vi "sub_pwrpak7_data-check.vi"() -> ()   [LabVIEW 2019]
panel:
  out "heading":dbl
  out "heading_check":bool
  out "heading_str":string
  out "index":i32
  out "경도":string="126.72082016226"
  out "위도":string="37.37012814476"
  out "utm-1":cluster{dbl, dbl}={530126.7583503594, 175270.68061157822} {"?" format="%#.6f"; "?" format="%.6f"}
  out "wgs84-1":cluster{dbl, dbl}={126.72082016226, 37.37012814476}
  in  "gps receive parsing array":string[](array[string])
  out "mode check":bool
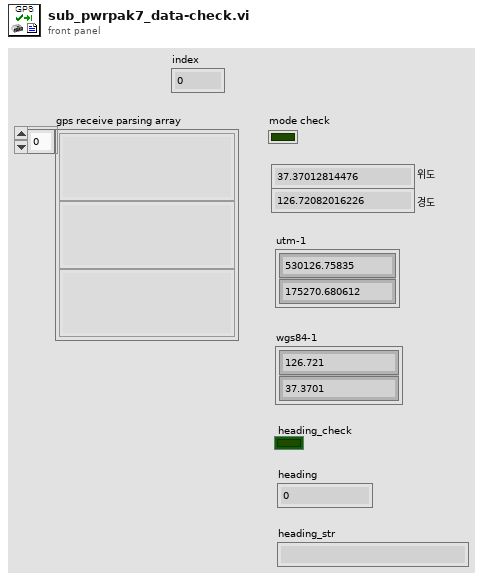
[diagram p1: front panel]
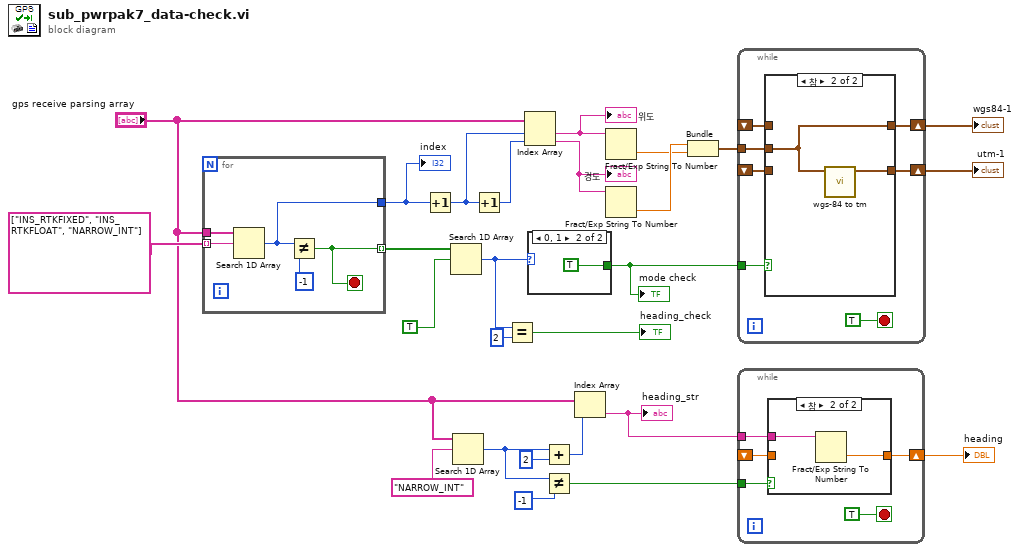
[diagram p0: block diagram]
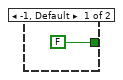
[diagram p2: hidden frame]
diagram:
  n1 = for {
    tunnel: [w28] -> w7 mode=indexing
    tunnel: "gps receive parsing array" -> [w31]
    tunnel: string[] ["INS_RTKFIXED", "INS_RTKFLOAT", "NARROW_INT"] -> [w29] mode=indexing
    tunnel: [w27] -> w17
    stop <- w28 stop-if-true
    n2 = Search 1D Array(1D array=w31, element=w29) -> (index of element=w27:i32)  [unwired: 1 in]
    n3 = Not Equal?(x=w27, y=-1) -> (x != y?=w28:bool)
  }
  "index" <- w17
  n4 = Increment(x=w17) -> (x+1=w21:i32)
  n5 = Search 1D Array(1D array=w7, element=TRUE ("원소")) -> (index of element=w3:i32)  [unwired: 1 in]
  n6 = Search 1D Array(1D array="gps receive parsing array", element="NARROW_INT" ("원소")) -> (index of element=w13:i32)  [unwired: 1 in]
  n7 = Increment(x=w21) -> (x+1=w20:i32)
  n8 = Equal?(x=w3, y=2) -> (x = y?=→"heading_check":bool)
  n9 = Index Array(array="gps receive parsing array", index #1=w21, index #2=w20) -> (element #1=w26:string, element #2=w25:string)
  "위도" <- w26
  "경도" <- w25
  n10 = case shown="0, 1" w3 {
    tunnel: [FALSE TRUE] -> w2
    frame -1, Default {
    }
    frame 0, 1 {
    }
  }
  "mode check" <- w2
  n11 = Add(x=w13, y=2) -> (x+y=w15:i32)
  n12 = Not Equal?(x=w13, y=-1) -> (x != y?=w10:bool)
  n13 = Index Array(array="gps receive parsing array", index=w15) -> (element=w9:string)
  "heading_str" <- w9
  n14 = Fract/Exp String To Number(string=w26) -> (number=w18:dbl)  [unwired: 3 in, 1 out]
  n15 = Fract/Exp String To Number(string=w25) -> (number=w19:dbl)  [unwired: 3 in, 1 out]
  n16 = Bundle(w19, w18) -> (w16:cluster{dbl, dbl})  [unwired: 1 in]
  n17 = while {
    tunnel: w2 -> [w39]
    shift-right: [w38] -> w22
    shift-left: _ -> [w36]
    shift-right: [w37] -> w23
    shift-left: _ -> [w35]
    tunnel: w16 -> [w34]
    stop <- TRUE stop-if-true
    n18 = case shown="참" w39 {
      tunnel: [w42 w43] -> w38
      tunnel: w34 -> [_ w43]
      tunnel: [w41 w44] -> w37
      tunnel: w36 -> [w42 _]
      tunnel: w35 -> [w41 _]
      frame False {
      }
      frame True {
        n19 = call "wgs-84 to tm.vi"("in_lon-lat"=w43) -> ("TM"=w44:cluster{"Y(E)":dbl, "X(N)":dbl})  [unwired: 10 in]
      }
    }
  }
  "wgs84-1" <- w22
  "utm-1" <- w23
  n20 = while {
    tunnel: w10 -> [w48]
    shift-right: [w46] -> w8
    shift-left: _ -> [w45]
    tunnel: w9 -> [w47]
    stop <- TRUE stop-if-true
    n21 = case shown="참" w48 {
      tunnel: w47 -> [_ w52]
      tunnel: [w50 w51] -> w46
      tunnel: w45 -> [w50 _]
      frame False {
      }
      frame True {
        n22 = Fract/Exp String To Number(string=w52) -> (number=w51:dbl)  [unwired: 3 in, 1 out]
      }
    }
  }
  "heading" <- w8
